vi "Write cell.vi"(8 "error in (no error)":errorcluster, 10 "cell":u8, 11 "Speaker Step in":refnum<class "Speaker Step.lvclass">) -> (0 "error out":errorcluster, 3 "Speaker Step out":refnum<class "Speaker Step.lvclass">)   [LabVIEW 2016, in "Controller.lvlib" / "Speaker Step.lvclass"]
uses:
  Speaker Step.lvclass
  Speaker Step.lvclass/Speaker Step.ctl
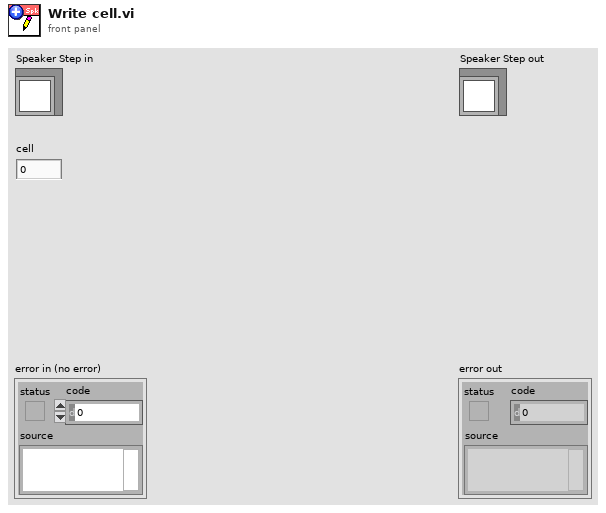
[diagram p1: front panel]
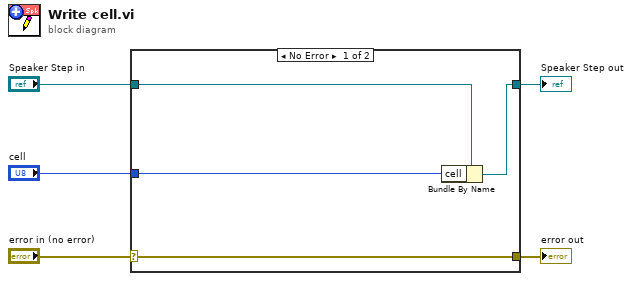
[diagram p0: block diagram]
diagram:
  n1 = case shown="No Error" "error in (no error)" {
    selector: "error in (no error)" -> [w9 w10]
    tunnel: [w9 w10] -> w4
    tunnel: [w7 w11] -> w2
    tunnel: "Speaker Step in" -> [w8 w11]
    tunnel: "cell" -> [w6 _]
    frame No Error {
      n2 = Bundle By Name(cluster=w8, "cell"=w6) -> (w7:refnum<class "Speaker Step.lvclass">)
    }
    frame Error {
    }
  }
  "error out" <- w4
  "Speaker Step out" <- w2
